vi "Msg.Init.vi"(8 "Error (in)":errorcluster, 11 "Queue Name (in)":string) -> (0 "Error (out)":errorcluster, 3 "Msg.Refs":T1)   [LabVIEW 2023]
doc: "This VI initializes all references for a given module."
uses:
  Msg.Data.ctl
  Msg.Q.Ref.ctl
  Msg.Event.Ref.ctl
  Msg.Event.RegRef.ctl
  Msg.Refs.ctl
  Msg.Noti.Ref.ctl
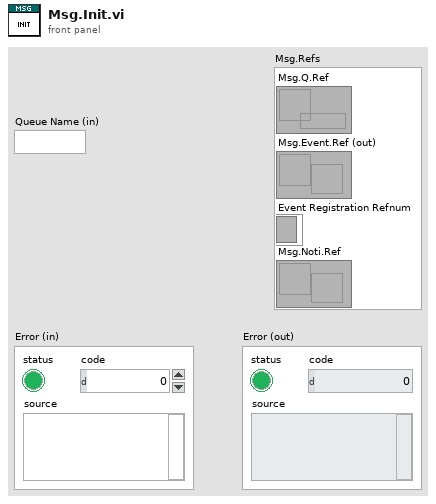
[diagram p1: front panel]
types:
  T1 = typedef "Msg.Refs.ctl" = cluster{"Msg.Q.Ref":T2, "Msg.Event.Ref (out)":T3, "Event Registration Refnum":T4, "Msg.Noti.Ref":T5}
  T2 = typedef "Msg.Q.Ref.ctl" = refnum<queue>
  T3 = typedef "Msg.Event.Ref.ctl" = refnum<user-event>
  T4 = typedef "Msg.Event.RegRef.ctl" = refnum<event-registration>
  T5 = typedef "Msg.Noti.Ref.ctl" = refnum<notifier>
  T6 = typedef "MessagingModule.lvlib/Msg.Refs.ctl" = cluster{"Msg.Q.Ref":T2, "Msg.Event.Ref (out)":T3, "Event Registration Refnum":T4, "Msg.Noti.Ref":T5}
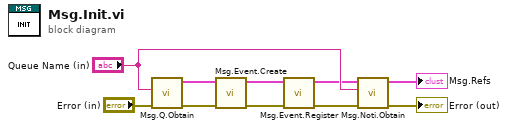
[diagram p0: block diagram]
diagram:
  n1 = call "Msg.Q.Obtain.vi"("Error (in)"="Error (in)", "Queue Name (in)"="Queue Name (in)") -> ("Error (out)"=w10:errorcluster, "Msg.Refs (out)"=w5:T6)  [unwired: 8 in]
  n2 = call "Msg.Event.Create.vi"("Error (in)"=w10, "Msg.Refs"=w5) -> ("Error (out)"=w9:errorcluster, "Msg.Refs (out)"=w4:T1)  [unwired: 8 in]
  n3 = call "Msg.Event.Register.vi"("Error (in)"=w9, "Msg.Refs"=w4) -> ("Error (out)"=w7:errorcluster, "Msg.Refs (out)"=w2:T1)  [unwired: 8 in]
  n4 = call "Msg.Noti.Obtain.vi"("error in (no error)"=w7, "Notifier Name"="Queue Name (in)", "Msg.Refs"=w2) -> ("error out"=→"Error (out)":errorcluster, "Msg.Refs (out)"=→"Msg.Refs":T1)  [unwired: 7 in]
